vi "StartStopDO.vi"(0 "object in":refnum<class "AD2_DO_SDK.lvclass">, 2 "Running":bool, 5 "error in (no error)":errorcluster) -> (14 "object out":refnum<class "AD2_DO_SDK.lvclass">, 19 "error out":errorcluster)   [LabVIEW 2021, in "AD2_DO_SDK.lvclass"]
uses:
  AD2_DO_SDK.lvclass
  AD2_DO_SDK.lvclass/AD2_DO_SDK.ctl
  Olasdwf/Olasdwf.lvlib
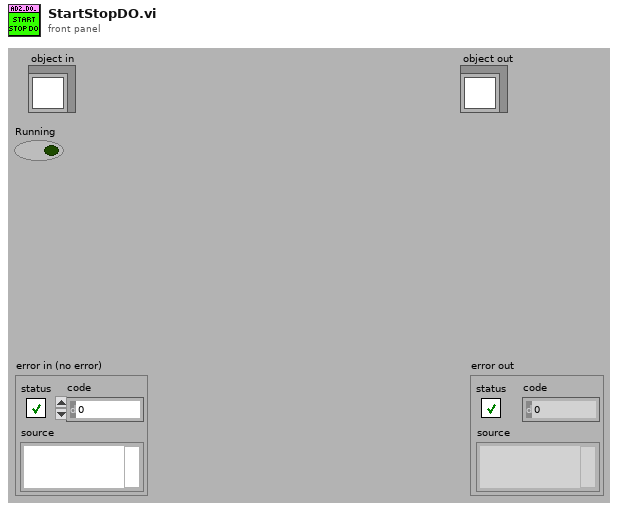
[diagram p1: front panel]
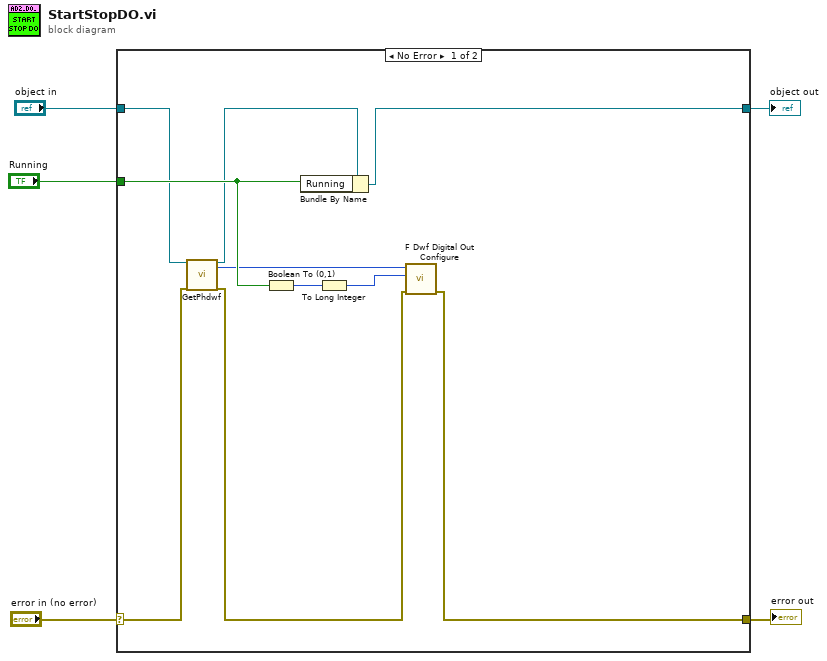
[diagram p0: block diagram]
diagram:
  n1 = case shown="No Error" "error in (no error)" {
    selector: "error in (no error)" -> [w7 w17]
    tunnel: [w11 w17] -> w4
    tunnel: [w15 w16] -> w2
    tunnel: "object in" -> [w9 w16]
    tunnel: "Running" -> [w14 _]
    frame No Error {
      n2 = call-dynamic "GetPhdwf.vi"("object in"=w9, "error in (no error)"=w7) -> ("object out"=w10:refnum<class "AD2_DO_SDK.lvclass">, "phdwf"=w8:i32, "error out"=w6:errorcluster)  [unwired: 15 in]
      n3 = Boolean To (0,1)(Boolean=w14) -> (0, 1=w12:i16)
      n4 = Bundle By Name(cluster=w10, "Running"=w14) -> (w15:refnum<class "AD2_DO_SDK.lvclass">)
      n5 = To Long Integer(number=w12) -> (32bit integer=w13:i32)
      n6 = call "F Dwf Digital Out Configure.vi"("error in (no error)"=w6, "fStart"=w13, "hdwf"=w8) -> ("error out"=w11:errorcluster)  [unwired: 7 in, 1 out]
    }
    frame Error {
    }
  }
  "error out" <- w4
  "object out" <- w2
